vi "IsSearchGoalNode.vi"(8 "error in (no error)":errorcluster, 10 "NodeToIdentify in":refnum<data-value>, 11 "PathTree in":refnum<class "RouteTree.lvclass">) -> (0 "error out":errorcluster, 1 "IsNode":bool, 2 "NodeToIdentify out":refnum<data-value>, 3 "PathTree out":refnum<class "RouteTree.lvclass">)   [LabVIEW 2014, in "RouteTree.lvclass"]
uses:
  <userlib>/AdvancedDataStructures/ClassBased/Applications/RouteSearch/PathTree/RouteTree.lvclass
  <userlib>/AdvancedDataStructures/ClassBased/TreeNode/TreeNode.lvclass
  <userlib>/AdvancedDataStructures/ClassBased/Applications/RouteSearch/Waypoint/Waypoint.lvclass
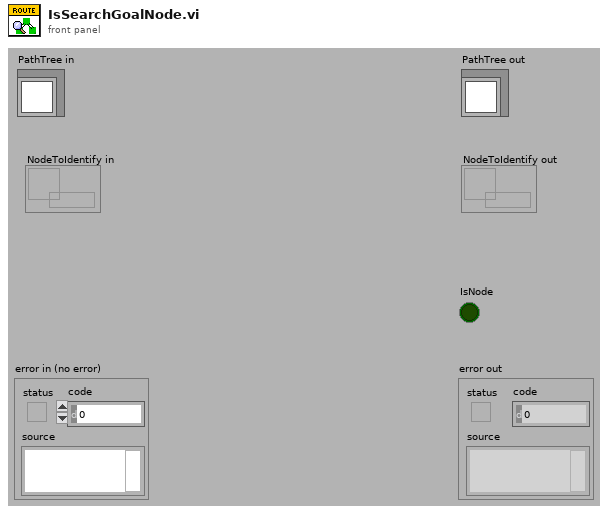
[diagram p1: front panel]
types:
  T1 = typedef "Waypoint.lvclass/point.ctl" = cluster{"X":dbl, "Y":dbl}
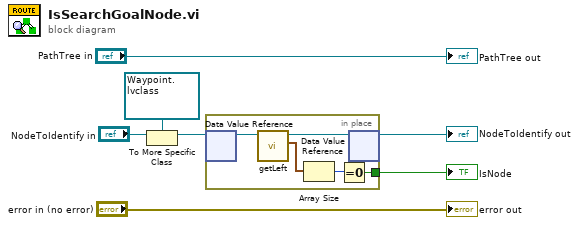
[diagram p0: block diagram]
diagram:
  n1 = To More Specific Class(target class=refnum<data-value> refnum ("data value reference"), reference="NodeToIdentify in") -> (specific class reference=w4:refnum<data-value>)  [unwired: 1 in, 1 out]
  n2 = in-place {
    in-place-border: [w8] -> w3
    n3 = in-place-dvr #1(w4) -> (w12:refnum<class "Waypoint.lvclass">)  [unwired: 1 out]
    n4 = call <userlib>:"getLeft.vi"("Waypoint in"=w12) -> ("left"=w10:T1[], "Waypoint out"=w11:refnum<class "Waypoint.lvclass">)  [unwired: 8 in, 1 out]
    n5 = Array Size(array=w10) -> (size(s)=w9:i32)
    n6 = Equal To 0?(x=w9) -> (x = 0?=w8:bool)
    n7 = in-place-dvr #1(w11) -> (→"NodeToIdentify out":refnum<data-value>)  [unwired: 1 out]
  }
  "IsNode" <- w3
  "error out" <- "error in (no error)"
  "PathTree out" <- "PathTree in"
